vi "Get Parameter (as Single).vi"(8 "error in (no error)":errorcluster, 10 "Parameter":T1, 11 "Sensor General Class in":refnum<class "Sensor General Class.lvclass">) -> (0 "error out":errorcluster, 2 "Data":sgl, 3 "Sensor General Class out":refnum<class "Sensor General Class.lvclass">)   [LabVIEW 2020, in "Sensor General Class.lvclass"]
uses:
  Sensor General Class.lvclass
  Parameters Enum.ctl
  Sensor General Class.lvclass/Sensor General Class.ctl
  <vilib>/NI Modbus.llb/MB Serial Master Query Read Holding Registers (poly).vi
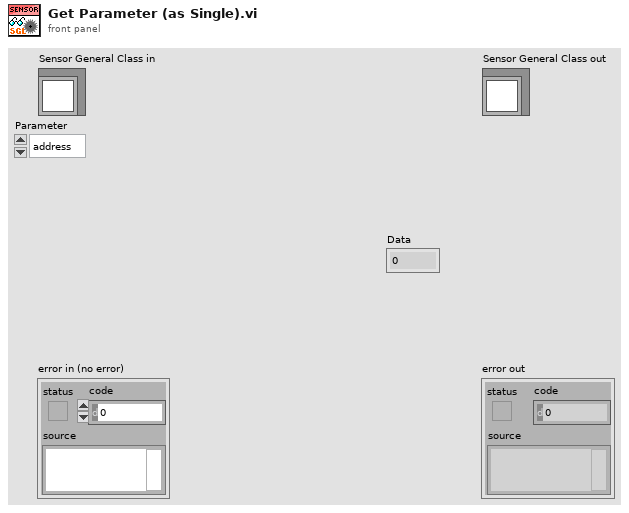
[diagram p1: front panel]
types:
  T1 = typedef "Sensor General Class.lvclass/Parameters Enum.ctl" = enum16{"address", "baud rate", "parity check", "load", "insulating gas", "additional component", "s/n", "hardware version", "firmware version", "humidity enable", "tag", "pressure offset", "humidity offset", "temperature offset", "service code"}
  T2 = cluster{"Mode":enum16{"RTU", "ASCII"}, "Slave Address":u8}
  T3 = cluster{"index":i32, "name":string, "register":u16, "word count":u16, "Write":bool}[]
  T4 = cluster{"index":i32, "name":string, "register":u16, "word count":u16, "Write":bool}
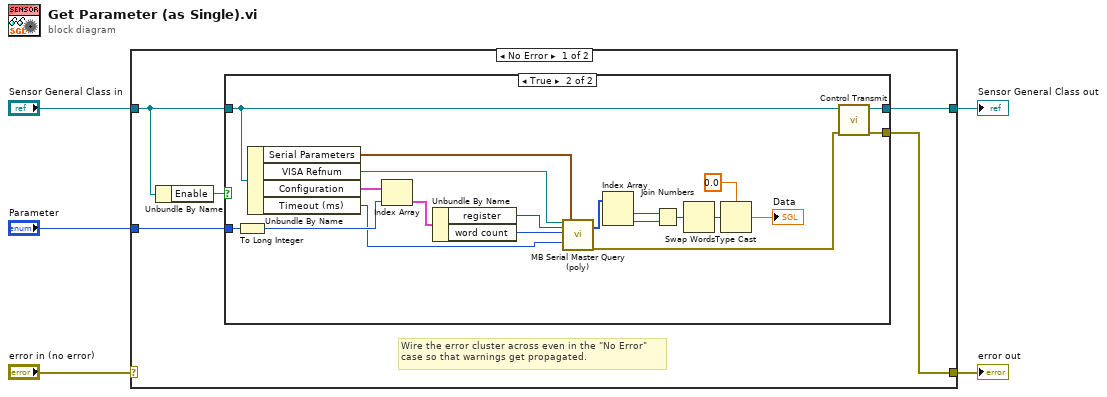
[diagram p0: block diagram]
diagram:
  n1 = case shown="No Error" "error in (no error)" {
    selector: "error in (no error)" -> [_ w33]
    tunnel: [w8 w33] -> w4
    tunnel: [w9 w32] -> w2
    tunnel: "Sensor General Class in" -> [w6 w32]
    tunnel: "Parameter" -> [w10 _]
    frame No Error {
      # "Wire the error cluster across even in the \"No Error\"\ncase so that warnings get propagated."
      n2 = Unbundle By Name(w6) -> ("Enable"=w7:bool)
      n3 = case shown="True" w7 {
        tunnel: w10 -> [_ w23]
        tunnel: w6 -> [w11 w15]
        tunnel: [w11 w14] -> w9
        tunnel: [_ w12] -> w8
        frame False {
        }
        frame True {
          n4 = To Long Integer(number=w23) -> (32bit integer=w28:i32)
          n5 = Unbundle By Name(w15) -> ("Serial Parameters"=w31:T2, "VISA Refnum"=w30:refnum<visa-resource-name>, "Configuration"=w29:T3, "Timeout (ms)"=w25:u32)
          n6 = Index Array(array=w29, index=w28) -> (element=w27:T4)
          n7 = Unbundle By Name(w27) -> ("register"=w26:u16, "word count"=w24:u16)
          n8 = call-poly <vilib>:"MB Serial Master Query (poly).vi"("VISA resource name"=w30, "Starting Address"=w26, "Quantity"=w24, "Timeout"=w25, "Serial Parameters"=w31) -> ("Holding Registers"=w17:u16[], "error out"=w13:errorcluster)  [unwired: 11 in, 2 out]
          n9 = Index Array(array=w17) -> (element #1=w18:u16, element #2=w16:u16)  [unwired: 2 in]
          n10 = Join Numbers(hi=w18, lo=w16) -> ((hi.lo)=w22:u32)
          n11 = Swap Words(1:w22) -> (0:w21:u32)
          n12 = Type Cast(type=sgl 0.0 ("p_atm"), x=w21) -> (*(type *) &x=→"Data":sgl)
          n13 = call-dynamic "Control Transmit.vi"("error in (no error)"=w13, "Sensor General Class in"=w15) -> ("error out"=w12:errorcluster, "Sensor General Class out"=w14:refnum<class "Sensor General Class.lvclass">)  [unwired: 8 in]
        }
      }
    }
    frame Error {
    }
  }
  "error out" <- w4
  "Sensor General Class out" <- w2
